vi "tauSaturation.vi"(3 "N":dbl format="%.2f", 4 "Y":dbl format="%.2f", 5 "X":dbl format="%.2f") -> (0 "Nout":dbl, 1 "Yout":dbl, 2 "Xout":dbl)   [LabVIEW 2014]
uses:
  <vilib>/imath/engines/lvmath2/RunTimeEngine/BuiltInFunctions/cos/NIMS_cos(C).vi
  <instcachedir>/0/NIMS_cos(C)_ED012A59E15C42DE86A4D91FD06B1A7E.lvgen/NIMS_cos(C)_ED012A59E15C42DE86A4D91FD06B1A7E_001.vi
  <vilib>/imath/engines/lvmath2/RunTimeEngine/BuiltInFunctions/sin/NIMS_sin(C).vi
  <instcachedir>/0/NIMS_sin(C)_7DEE2CE4F8924451850C309C60B7EC26.lvgen/NIMS_sin(C)_7DEE2CE4F8924451850C309C60B7EC26_001.vi
  <vilib>/imath/engines/lvmath2/RunTimeEngine/NodeEndStatement/NIMS_NodeEndStatement_Output.vi
  <instcachedir>/0/NIMS_NodeEndStatement_Output_53EC0D466D134D7ABD903AC30B43404B.lvgen/NIMS_NodeEndStatement_Output_53EC0D466D134D7ABD903AC30B43404B_010.vi
  <vilib>/imath/engines/lvmath2/RunTimeEngine/ErrorHandling/NIMS_Finalize Error.vi
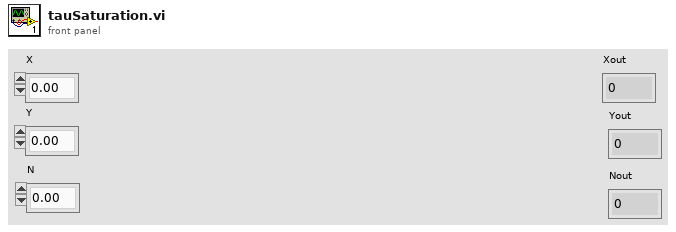
[diagram p1: front panel]
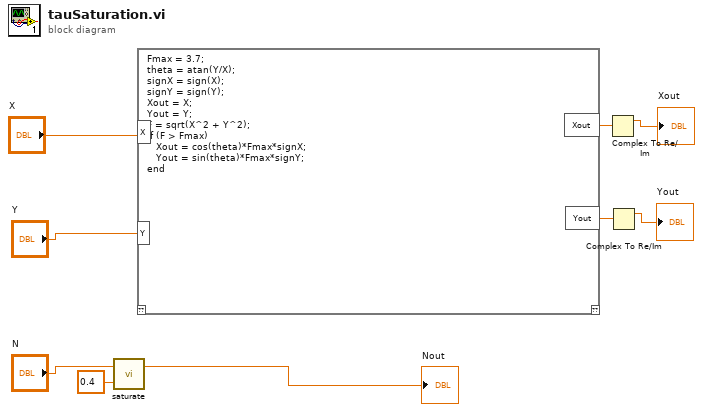
[diagram p0: block diagram]
diagram:
  n1 = call "saturate.vi"("amplitude"=0.4, "value"="N") -> ("saturated"=→"Nout":dbl)  [unwired: 1 out]
  n2 = mathscript code="Fmax = 3.7;\ntheta = atan(Y/X);\nsignX = sign(X);\nsignY = sign(Y);\nXout = X;\nYout = Y;\nF = sqrt(X^2 + Y^2);\nif (F > Fmax)\n   Xout = cos(theta)*Fmax*signX;\n   Yout = sin(theta)*Fmax*signY;\nend"("X"="X", "Y"="Y") -> ("Xout"=w2:cdb, "Yout"=w4:cdb)  [unwired: 1 in, 1 out]
  n3 = Complex To Re/Im(x + iy=w2) -> (x=→"Xout":dbl)  [unwired: 1 out]
  n4 = Complex To Re/Im(x + iy=w4) -> (x=→"Yout":dbl)  [unwired: 1 out]
